vi "Test or run batch file.vi"(7 "Cmd string (to log)":string="test fieldscan_up.txt", 8 "error in":errorcluster caption="error in (no error)", 10 "Action":T1, 11 "Batch file path":path=path "D:/ACM in LabVIEW/_batch (NIW test)/fieldscan_up.txt") -> (0 "error out":errorcluster, 1 "Cmds array":string[](array[string]))   [LabVIEW 2019]
doc: "Nicolas Weiss - EPFL - IPHYS 2019\n----\nThis VI \"test\" or \"run\" a batch file located in the \"Batch file directory\" define in the LabVIEW \"Global variable 1.vi\"\n\nThis VI parses the batch commands (line by line) and creates an array of those commands.\nThis array is sent to the \"Check and send\" command."
uses:
  Controls/Test-run selector.ctl
  Controls/Log destination selector.ctl
  <vilib>/Utility/file.llb/Read Delimited Spreadsheet (string).vi
  _Global variables 1.vi
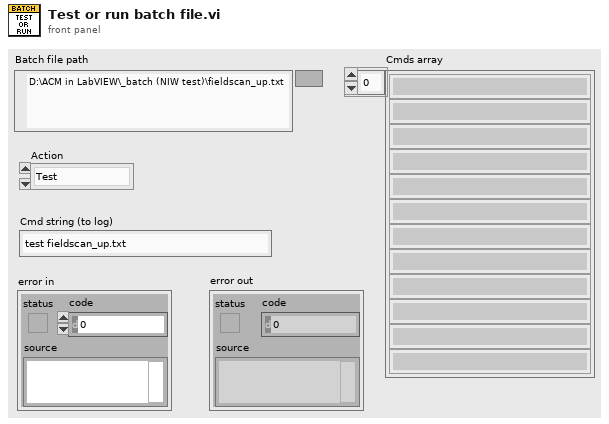
[diagram p1: front panel]
types:
  T1 = typedef "Test-run selector.ctl" = enum16{"Test", "Run"}
  T2 = typedef "Log destination selector.ctl" = enum16{"UI", "File", "UI+file"}
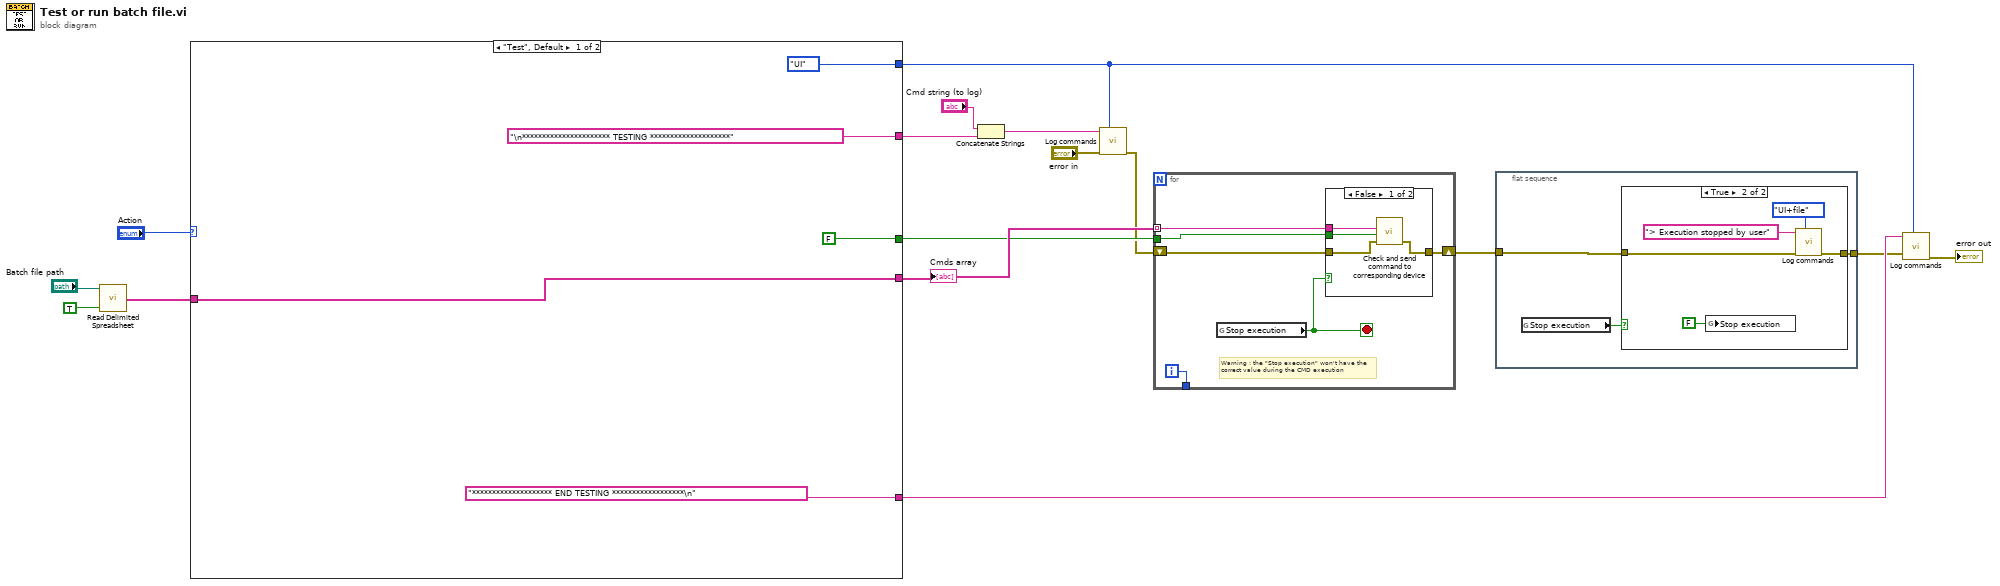
[diagram p0: block diagram]
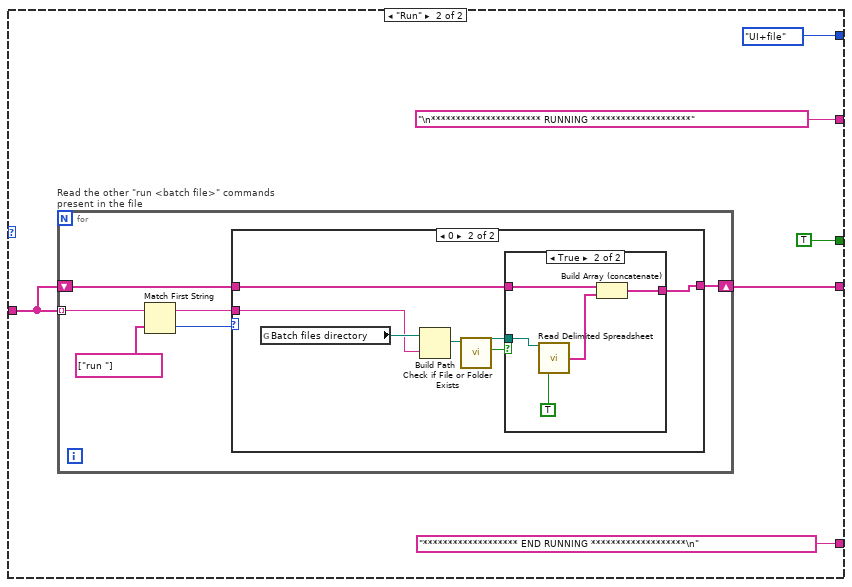
[diagram p3: hidden frame]
diagram:
  n1 = call-poly <vilib>:"Read Delimited Spreadsheet.vi"("file path (dialog if empty)"="Batch file path", "transpose? (F)"=TRUE) -> ("first row"=w14:string[])  [unwired: 8 in, 5 out]
  n2 = case shown="\"Test\", Default" "Action" {
    tunnel: w14 -> [w21 w25]
    tunnel: [w21 w24] -> w12
    tunnel: ["\n********************** TESTING ********************" ("text to log") "\n********************** RUNNING ********************" ("text to log")] -> w10
    tunnel: ["******************** END TESTING ******************\n" ("text to log") "******************* END RUNNING *******************\n" ("text to log")] -> w3
    tunnel: [FALSE ("Log cmd (T)") TRUE ("Log cmd (T)")] -> w11
    tunnel: [Log_destination_selector."UI" ("Log destination") Log_destination_selector."UI+file" ("Log destination")] -> w4
    frame "Test", Default {
    }
    frame "Run" {
      n3 = for "Read the other \"run <batch file>\" commands present in the file" {
        tunnel: w25 -> [w33] mode=indexing
        shift-right: [w28] -> w24
        shift-left: w25 -> [w30]
        n4 = Match First String(2:string[] ["run "] ("string array"), 3:w33) -> (0:w31:i32, 1:w29:string)
        n5 = case shown="0" w31 {
          tunnel: w30 -> [w34 w37]
          tunnel: w29 -> [_ w39]
          tunnel: [w34 w35] -> w28
          frame Default {
          }
          frame 0 {
            n6 = global read "_Global variables 1.vi" "Batch files directory"() -> (w40:path)
            n7 = Build Path(base path=w40, name or relative path=w39) -> (appended path=w41:path)
            n8 = call <vilib>:"Check if File or Folder Exists.vi"("path"=w41) -> ("file or folder exists?"=w38:bool, "dup path"=w36:path)  [unwired: 8 in, 1 out]
            n9 = case shown="True" w38 {
              tunnel: w37 -> [w42 w45]
              tunnel: w36 -> [_ w46]
              tunnel: [w42 w43] -> w35
              frame False {
              }
              frame True {
                n10 = call-poly <vilib>:"Read Delimited Spreadsheet.vi"("file path (dialog if empty)"=w46, "transpose? (F)"=TRUE) -> ("first row"=w44:string[])  [unwired: 8 in, 5 out]
                n11 = Build Array (concatenate)(w45, w44) -> (w43:string[])
              }
            }
          }
        }
      }
    }
  }
  "Cmds array" <- w12
  n12 = Concatenate Strings("Cmd string (to log)", w10) -> (w6:string)
  n13 = call "Log commands.vi"("Log destination"=w4, "error in"="error in", "text to log"=w6) -> ("error out"=w7:errorcluster)  [unwired: 8 in]
  n14 = for {
    tunnel: w12 -> [w53] mode=indexing
    tunnel: w11 -> [w50]
    shift-right: [w51] -> w2
    shift-left: w7 -> [w52]
    tunnel: [w48] -> _
    i -> [w48]
    stop <- w49 stop-if-true
    # "Warning : the \"Stop execution\" won't have the\ncorrect value during the CMD execution"
    n15 = global read "_Global variables 1.vi" "Stop execution"() -> (w49:bool)
    n16 = case shown="False" w49 {
      tunnel: w53 -> [w57 _]
      tunnel: w52 -> [w56 w58]
      tunnel: [w55 w58] -> w51
      tunnel: w50 -> [w54 _]
      frame False {
        n17 = call "Check and send command to corresponding device.vi"("error in (no error)"=w56, "Execute cmd (F)"=w54, "Cmd string"=w57) -> ("error out"=w55:errorcluster)  [unwired: 7 in, 1 out]
      }
      frame True {
      }
    }
  }
  n18 = flat-sequence {
    tunnel: w2 -> [w61]
    tunnel: [w60] -> w1
    frame #0 {
      n19 = global read "_Global variables 1.vi" "Stop execution"() -> (w59:bool)
      n20 = case shown="True" w59 {
        tunnel: w61 -> [w62 w65]
        tunnel: [w62 w64] -> w60
        frame False {
        }
        frame True {
          n21 = global write "_Global variables 1.vi" "Stop execution"(FALSE ("Stop execution")) -> ()
          n22 = call "Log commands.vi"("Log destination"=Log_destination_selector."UI+file", "error in"=w65, "text to log"="> Execution stopped by user") -> ("error out"=w64:errorcluster)  [unwired: 8 in]
        }
      }
    }
  }
  n23 = call "Log commands.vi"("Log destination"=w4, "error in"=w1, "text to log"=w3) -> ("error out"=→"error out":errorcluster)  [unwired: 8 in]
